vi "主.vi"() -> ()   [LabVIEW 2016]
panel:
  in  "删除按钮":bool
  in  "添加按钮":bool
  in  "选项卡控件":T1(tab)
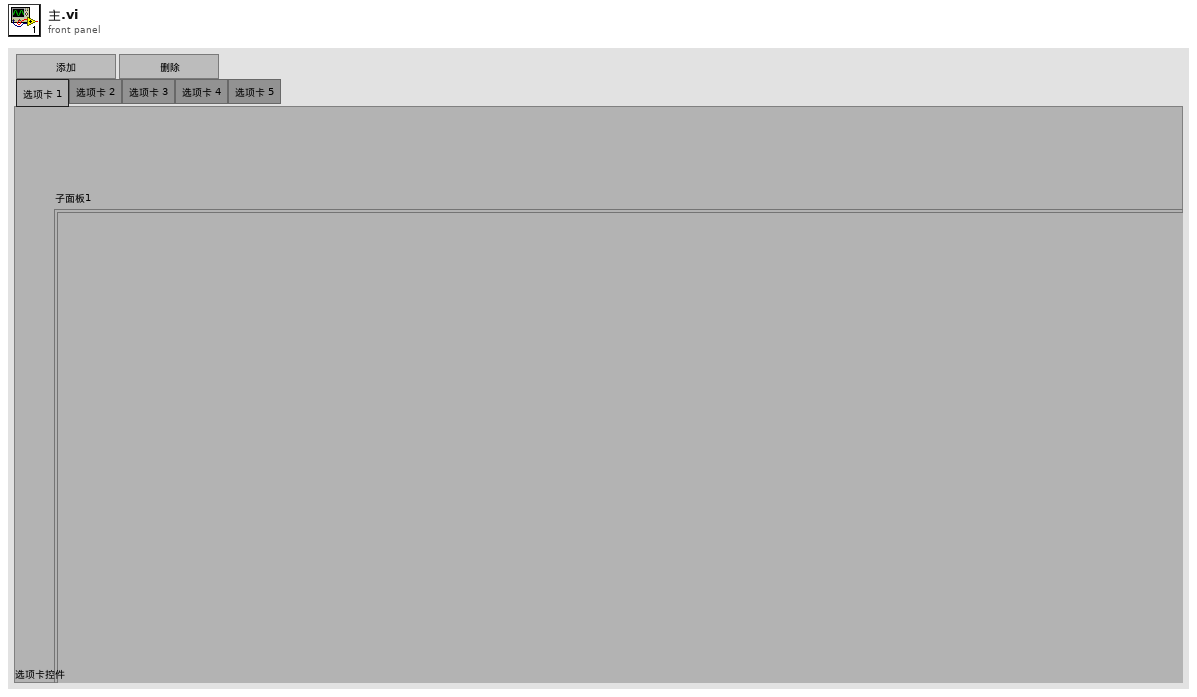
[diagram p1: front panel]
types:
  T1 = enum32{"选项卡 1", "选项卡 2", "选项卡 3", "选项卡 4", "选项卡 5"}
  T2 = typedef "imagedata.ctl" = cluster{"image type":i32, "image depth":i32, "image":u8[], "mask":u8[], "colors":u32[], "Rectangle":cluster{"left":i16, "top":i16, "right":i16, "bottom":i16}}
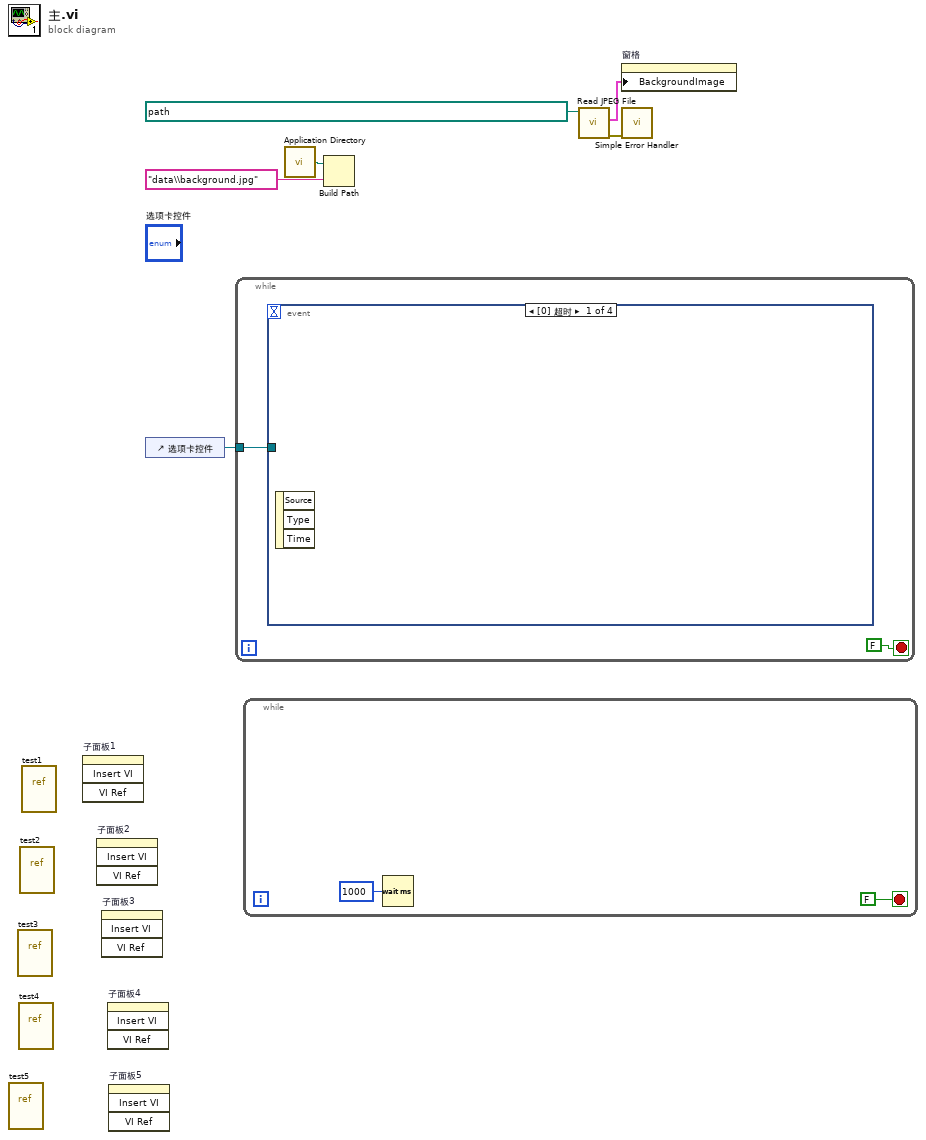
[diagram p0: block diagram]
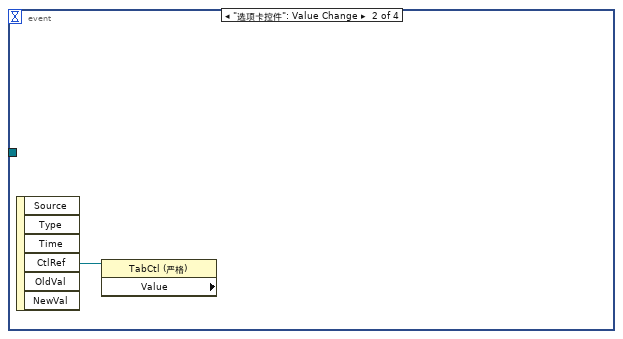
[diagram p2: hidden frame]
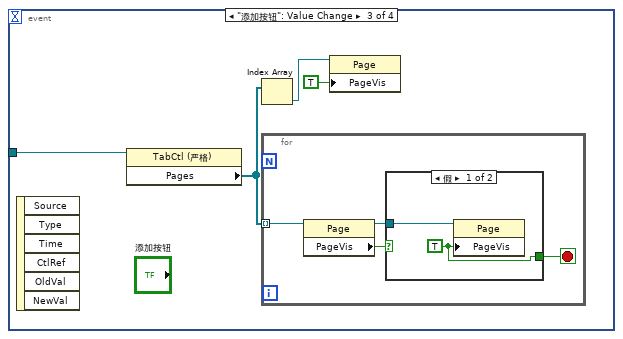
[diagram p3: hidden frame]
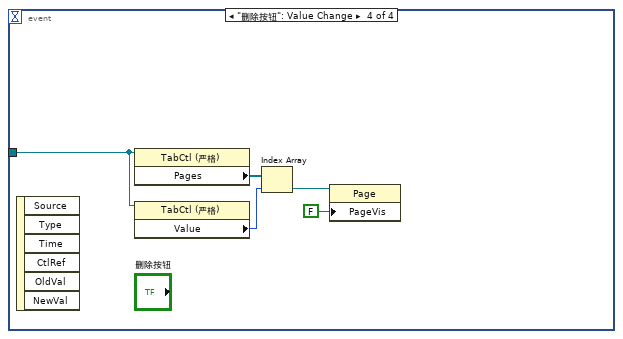
[diagram p5: hidden frame]
diagram:
  n1 = vi-ref "test5.vi"() -> ()  [unwired: 1 out]
  n2 = vi-ref "test3.vi"() -> ()  [unwired: 1 out]
  n3 = vi-ref "test4.vi"() -> ()  [unwired: 1 out]
  n4 = vi-ref "test2.vi"() -> ()  [unwired: 1 out]
  n5 = vi-ref "test1.vi"() -> ()  [unwired: 1 out]
  n6 = invoke on="子面板1" class="SubPnl" method="Insert VI"() -> ()  [unwired: 4 in, 4 out]
  n7 = invoke on="子面板2" class="SubPnl" method="Insert VI"() -> ()  [unwired: 4 in, 4 out]
  n8 = invoke on="子面板3" class="SubPnl" method="Insert VI"() -> ()  [unwired: 4 in, 4 out]
  n9 = invoke on="子面板4" class="SubPnl" method="Insert VI"() -> ()  [unwired: 4 in, 4 out]
  n10 = invoke on="子面板5" class="SubPnl" method="Insert VI"() -> ()  [unwired: 4 in, 4 out]
  n11 = control-ref of="选项卡控件"() -> (w1:refnum<vi>)
  n12 = while {
    tunnel: w1 -> [w7]
    stop <- FALSE stop-if-true
    n13 = event shown="[0] 超时" {
      selector: _ -> [_ _ _ _]
      dyn-events: _ -> [_ _ _ _]
      timeout: _ -> [_ _ _ _]
      tunnel: w7 -> [_ _ w11 w21]
      event Timeout {
        n14 = event-data() -> ()  [unwired: 1 in, 3 out]
      }
      event "选项卡控件": Value Change {
        n15 = event-data() -> ("CtlRef"=w9:refnum<vi>)  [unwired: 1 in, 5 out]
        n16 = property class="TabCtl (严格)" props=["Value"](reference=w9) -> ()  [unwired: 1 in, 3 out]
      }
      event "添加按钮": Value Change {
        n17 = event-data() -> ()  [unwired: 1 in, 6 out]
        n18 = property class="TabCtl (严格)"(reference=w11) -> ("Pages"=w10:refnum<vi>[])  [unwired: 1 in, 2 out]
        n19 = Index Array(array=w10) -> (element=w13:refnum<vi>)  [unwired: 1 in]
        n20 = for {
          tunnel: w10 -> [w17] mode=indexing
          stop <- w15 stop-if-true
          n21 = property class="Page"(reference=w17) -> (reference out=w14:refnum<vi>, "PageVis"=w16:bool)  [unwired: 1 in, 1 out]
          n22 = case shown="假" w16 {
            tunnel: [w19 _] -> w15
            tunnel: w14 -> [w18 _]
            frame False {
              w19 = TRUE ("选项卡可见")
              n23 = property class="Page"(reference=w18, "PageVis"=w19) -> ()  [unwired: 1 in, 2 out]
            }
            frame True {
            }
          }
        }
        n24 = property class="Page"(reference=w13, "PageVis"=TRUE ("选项卡可见")) -> ()  [unwired: 1 in, 2 out]
      }
      event "删除按钮": Value Change {
        n25 = event-data() -> ()  [unwired: 1 in, 6 out]
        n26 = property class="TabCtl (严格)"(reference=w21) -> ("Pages"=w23:refnum<vi>[])  [unwired: 1 in, 2 out]
        n27 = property class="TabCtl (严格)"(reference=w21) -> ("Value"=w20:T1)  [unwired: 1 in, 2 out]
        n28 = Index Array(array=w23, index=w20) -> (element=w24:refnum<vi>)
        n29 = property class="Page"(reference=w24, "PageVis"=FALSE ("选项卡可见")) -> ()  [unwired: 1 in, 2 out]
      }
    }
  }
  n30 = while {
    stop <- FALSE stop-if-true
    n31 = Wait (ms)(milliseconds to wait=u32 1000 ("等待时间（毫秒）")) -> ()  [unwired: 1 out]
  }
  n32 = call <vilib>:"Application Directory.vi"() -> ("Application Directory"=w5:path)
  n33 = Build Path(base path=w5, name or relative path="data\\background.jpg" ("名称或相对路径")) -> ()  [unwired: 1 out]
  n34 = call <vilib>:"Read JPEG File.vi"("path to JPEG file"=path "F:/gitkraken/CC/平台数采程序 - V3（多开测试版）/data/background.jpg") -> ("error out"=w4:errorcluster, "image data"=w3:T2)  [unwired: 8 in, 1 out]
  n35 = property on="窗格" class="Pane"("BackgroundImage"=w3) -> ()  [unwired: 2 in, 2 out]
  n36 = call <vilib>:"Simple Error Handler.vi"("error in (no error)"=w4) -> ()  [unwired: 4 in, 5 out]
